vi "_attribute_write_rawstring.vi"(5 "Repeated Capability":string, 7 "Attribute":T1={"Identifier"="", "Descriptive Name"="", "Data Type"=enum."Integer 32", "Command"="", "Access"=enum."Read/Write", "Range Table"="", "Read Callback"="", "Write Callback"="", "Supported Models"="", "Instrument Options"="", "Index"=0, "OPC Wait"=FALSE, "No Status Check"=FALSE, "Cache Only"=FALSE}, 8 "error in":errorcluster caption="error in (no error)", 10 "Raw String in":string, 11 "VISA resource name":refnum<visa-resource-name>) -> (0 "error out":errorcluster, 3 "VISA resource name out":refnum<visa-resource-name>)   [LabVIEW 2020, in "Rohde&Schwarz RTx Oscilloscopes.lvlib" / "rsidr_core.lvlib"]
uses:
  rsidr_core.lvlib
  type_Attribute.ctl
  type_Attribute_Data_Type.ctl
  type_ReadWriteAccess.ctl
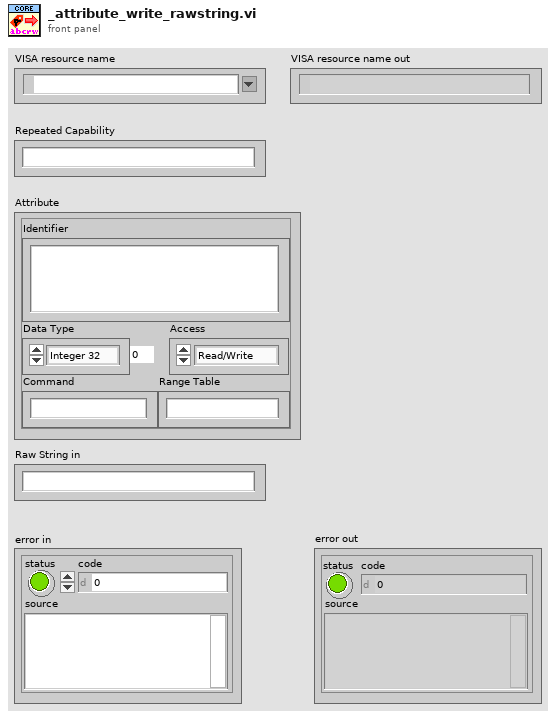
[diagram p1: front panel]
types:
  T1 = typedef "Rohde&Schwarz RTx Oscilloscopes.lvlib/rsidr_core.lvlib/type_Attribute.ctl" = cluster{"Identifier":string, "Descriptive Name":string, "Data Type":T2, "Command":string, "Access":T3, "Range Table":string, "Read Callback":string, "Write Callback":string, "Supported Models":string, "Instrument Options":string, "Index":i32, "OPC Wait":bool, "No Status Check":bool, "Cache Only":bool}
  T2 = typedef "Rohde&Schwarz RTx Oscilloscopes.lvlib/rsidr_core.lvlib/type_Attribute_Data_Type.ctl" = enum16{"Integer 32", "Double", "String", "Boolean", "None", "Integer 64", "RawString"}
  T3 = typedef "Rohde&Schwarz RTx Oscilloscopes.lvlib/rsidr_core.lvlib/type_ReadWriteAccess.ctl" = enum16{"Read Only", "Write Only", "Read/Write"}
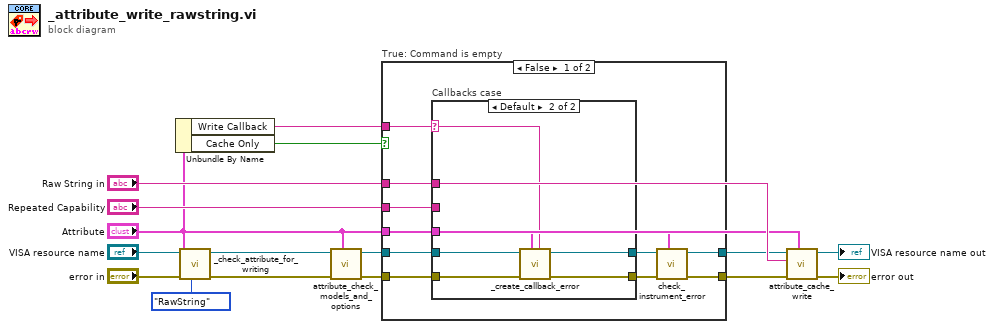
[diagram p0: block diagram]
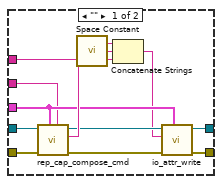
[diagram p2: hidden frame]
diagram:
  n1 = Unbundle By Name("Attribute") -> ("Write Callback"=w9:string, "Cache Only"=w1:bool)
  n2 = call "_check_attribute_for_writing.vi"("Expected Data Type"=type_Attribute_Data_Type."RawString" ("Data Type"), "Attribute"="Attribute", "error in"="error in", "VISA resource name"="VISA resource name") -> ("error out"=w8:errorcluster, "VISA resource name out"=w7:refnum<visa-resource-name>)  [unwired: 6 in]
  n3 = call "attribute_check_models_and_options.vi"("Attribute"="Attribute", "error in"=w8, "VISA resource name"=w7) -> ("error out"=w6:errorcluster, "VISA resource name out"=w5:refnum<visa-resource-name>)  [unwired: 6 in, 1 out]
  n4 = case "True: Command is empty" shown="False" w1 {
    tunnel: "Repeated Capability" -> [w26 _]
    tunnel: w6 -> [w23 w45]
    tunnel: w5 -> [w22 w46]
    tunnel: "Raw String in" -> [w25 _]
    tunnel: "Attribute" -> [w17 _]
    tunnel: [w18 w46] -> w3
    tunnel: [w19 w45] -> w4
    tunnel: w9 -> [w24 _]
    frame False {
      n5 = case "Callbacks case" shown="Default" w24 {
        selector: w24 -> [_ w39]
        tunnel: w25 -> [w29 _]
        tunnel: w22 -> [w36 w43]
        tunnel: w23 -> [w37 w44]
        tunnel: w26 -> [w30 _]
        tunnel: [w32 w41] -> w20
        tunnel: [w33 w42] -> w21
        tunnel: w17 -> [w31 w40]
        frame "" {
          n6 = call "rep_cap_compose_cmd.vi"("Repeated Capability"=w30, "Attribute"=w31, "error in"=w37, "VISA resource name"=w36) -> ("error out"=w35:errorcluster, "Command out"=w38:string, "VISA resource name out"=w34:refnum<visa-resource-name>)  [unwired: 5 in]
          n7 = call "Space Constant.vi"() -> ("String"=w27:string)
          n8 = Concatenate Strings(w38, w27, w29) -> (w28:string)
          n9 = call "io_attr_write.vi"("Attribute"=w31, "error in"=w35, "write buffer"=w28, "VISA resource name"=w34) -> ("error out"=w33:errorcluster, "VISA resource name out"=w32:refnum<visa-resource-name>)  [unwired: 6 in]
        }
        frame Default {
          n10 = call "_create_callback_error.vi"("Callback Name"=w39, "Attribute"=w40, "error in"=w44, "VISA resource name"=w43) -> ("error out"=w42:errorcluster, "VISA resource name out"=w41:refnum<visa-resource-name>)  [unwired: 6 in]
        }
      }
      n11 = call "check_instrument_error.vi"("Attribute"=w17, "error in"=w21, "VISA resource name"=w20) -> ("error out"=w19:errorcluster, "VISA resource name out"=w18:refnum<visa-resource-name>)  [unwired: 7 in]
    }
    frame True {
    }
  }
  n12 = call "attribute_cache_write.vi"("Attribute"="Attribute", "error in"=w4, "Value in"="Raw String in", "VISA resource name"=w3) -> ("error out"=→"error out":errorcluster, "VISA resource name out"=→"VISA resource name out":refnum<visa-resource-name>)  [unwired: 6 in]
